vi "EV Rotator Initialize.vi"(0 "Run Step Inputs":T1={"Data in"=[], "Results in"=[], "Seq Setup in"="", "Step name"="", "Hardware in"="", "Calibration in"="", "Step # in sequence"=0, "Display step?(f)"=TRUE, "Generate names only"=FALSE, "Waveforms in"=[], "Memory List Grouping info"=[]} {"Waveforms in"."Y dB ref" format="%.1f"; "Waveforms in"."Y axis" items=["dB", "Lin", "Pwr"]; "Waveforms in"."Y data" items=["dB", "Lin", "Pwr"]; "Waveforms in"."X data" items=["dB", "Lin", "Pwr"]; "Data in"."Z data" items=["dB", "Lin", "Pwr"]; "Data in"."X data" items=["dB", "Lin", "Pwr"]; "Data in"."Y data" items=["dB", "Lin", "Pwr"]; "Data in"."Z dB ref" format="%.1f"; "Data in"."Z axis" items=["Log", "Lin"]; "Data in"."X dB ref" format="%.1f"; "Data in"."X axis" items=["Log", "Lin"]; "Data in"."Y axis" items=["Log", "Lin"]; "Data in"."Y dB ref" format="%.1f"; "Data in"."Curve"."z" format="%.2f"; "Data in"."Curve"."y" format="%.2f"; "Data in"."Curve"."x" format="%.2f"; "Results in"."Unit type" items=["dB", "Lin", "Pwr"]; "Results in"."Margin" format="%.2f"}, 11 "error in (no error)":errorcluster) -> (6 "Data out":T2 {"Z data" items=["dB", "Lin", "Pwr"]; "X data" items=["dB", "Lin", "Pwr"]; "Y data" items=["dB", "Lin", "Pwr"]; "Z dB ref" format="%.1f"; "Z axis" items=["Log", "Lin"]; "X dB ref" format="%.1f"; "X axis" items=["Log", "Lin"]; "Y axis" items=["Log", "Lin"]; "Y dB ref" format="%.1f"; "Curve"."z" format="%.2f"; "Curve"."y" format="%.2f"; "Curve"."x" format="%.2f"}, 8 "Results out":T5 {"Unit type" items=["dB", "Lin", "Pwr"]; "Margin" format="%.2f"}, 10 "Waveforms out":T7 {"Y dB ref" format="%.1f"; "Y axis" items=["dB", "Lin", "Pwr"]; "Y data" items=["dB", "Lin", "Pwr"]; "X data" items=["dB", "Lin", "Pwr"]}, 15 "error out":errorcluster)   [LabVIEW 2016]
uses:
  custom and Sc run Seq Sub VIs (x64).llb/data array.ctl
  custom and Sc run Seq Sub VIs (x64).llb/data cluster.ctl
  custom and Sc run Seq Sub VIs (x64).llb/Axis Unit Type.ctl
  custom and Sc run Seq Sub VIs (x64).llb/result array.ctl
  custom and Sc run Seq Sub VIs (x64).llb/result cluster.ctl
  custom and Sc run Seq Sub VIs (x64).llb/waveform array.ctl
  custom and Sc run Seq Sub VIs (x64).llb/waveform cluster.ctl
  custom and Sc run Seq Sub VIs (x64).llb/Run Step Inputs.ctl
  custom and Sc run Seq Sub VIs (x64).llb/Memory List Grouping.ctl
  custom and Sc run Seq Sub VIs (x64).llb/Memory List Grouping - Item Type.ctl
  custom and Sc run Seq Sub VIs (x64).llb/window stack manager Functions.ctl
  C:/SoundCheck 17/System/Custom VIs/EV.Rotator.RotatorControl.dll
  EV.Rotator.RotatorControl.dll
panel:
  # "NOTE:  These controls and indicators must stay here, but you can Hide them if you wish.  These are wired as the standard input/output connector pane for step run VIs."
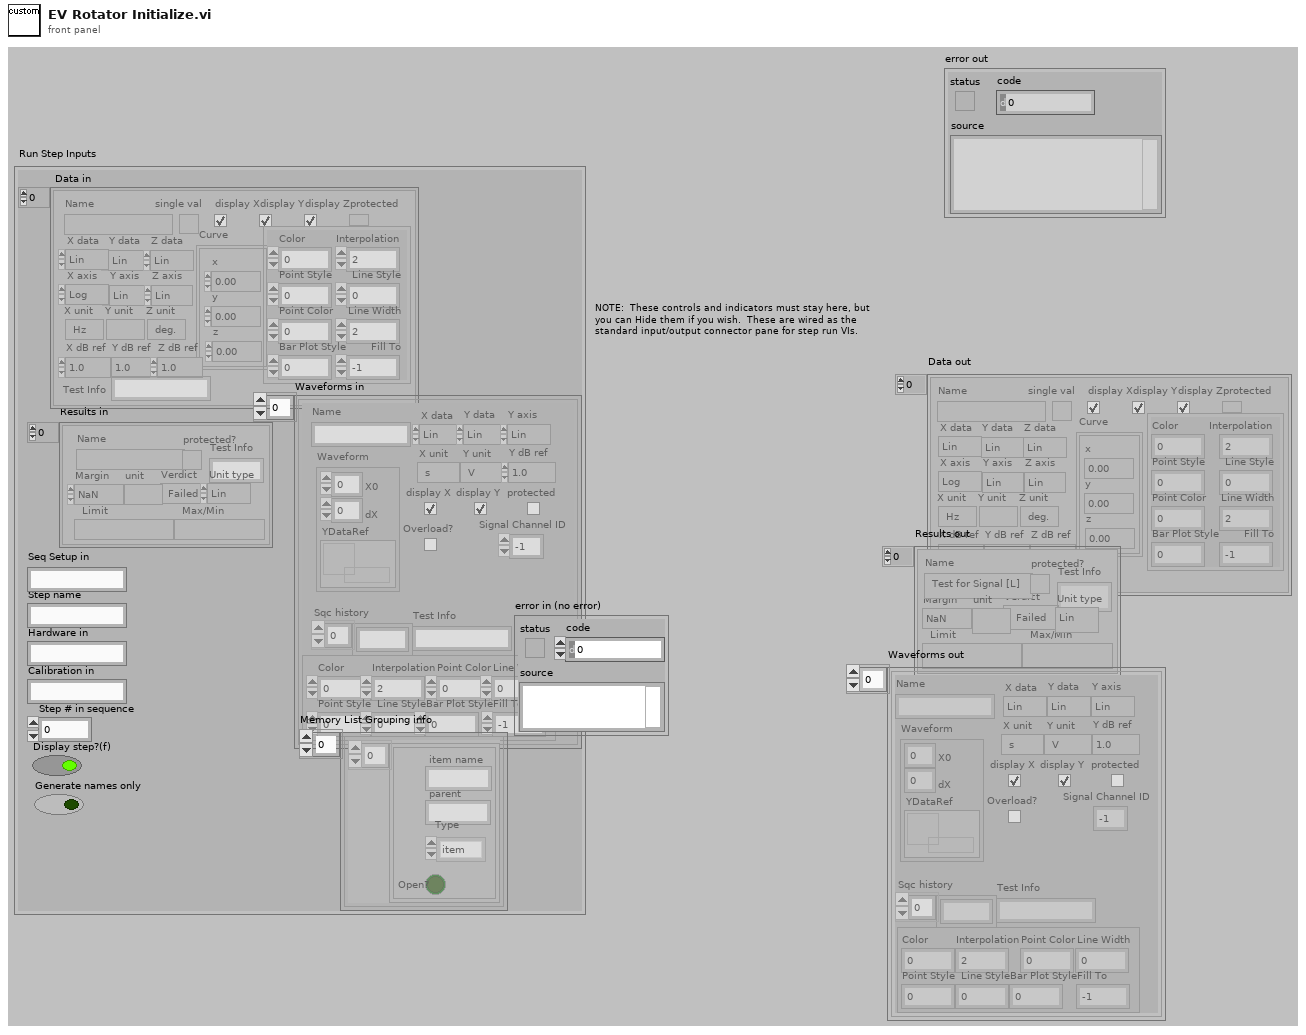
[diagram p1: front panel]
types:
  T1 = typedef "Run Step Inputs.ctl" = cluster{"Data in":T2, "Results in":T5, "Seq Setup in":string, "Step name":string, "Hardware in":string, "Calibration in":string, "Step # in sequence":i32, "Display step?(f)":bool, "Generate names only":bool, "Waveforms in":T7, "Memory List Grouping info":cluster{T9[]}[]}
  T2 = typedef "data array.ctl" = T3[]
  T3 = typedef "data cluster.ctl" = cluster{"Name":string, "Curve":cluster{"x":dbl, "y":dbl, "z":dbl}[], "X data":T4, "Y data":T4, "Z data":T4, "X axis":u16, "Y axis":u16, "Z axis":u16, "X unit":string, "Y unit":string, "Z unit":string, "X dB ref":dbl, "Y dB ref":dbl, "Z dB ref":dbl, "single val":bool, "protected":bool, "display X":bool, "display Y":bool, "display Z":bool, "Plot Settings":cluster{"Color":u32, "Interpolation":u8, "Point Style":u8, "Line Style":u8, "Point Color":u32, "Line Width":u8, "Bar Plot Style":u8, "Fill To":i16}, "Test Info":string}
  T4 = typedef "Axis Unit Type.ctl" = u16
  T5 = typedef "result array.ctl" = T6[]
  T6 = typedef "result cluster.ctl" = cluster{"Name":string, "Margin":dbl, "unit":string, "Verdict":bool, "Limit":string, "Max/Min":string, "protected?":bool, "Test Info":string, "Unit type":T4}
  T7 = typedef "waveform array.ctl" = T8[]
  T8 = typedef "waveform cluster.ctl" = cluster{"Name":string, "Waveform":cluster{"X0":dbl, "dX":dbl, "YDataRef":refnum<data-value>}, "X data":T4, "Y data":T4, "Y axis":T4, "X unit":string, "Y unit":string, "Y dB ref":dbl, "display Y":bool, "display X":bool, "Overload?":bool, "protected":bool, "Sqc history":string[], "Signal Channel ID":i32, "Plot Settings":cluster{"Color":u32, "Interpolation":u8, "Point Style":u8, "Line Style":u8, "Point Color":u32, "Line Width":u8, "Bar Plot Style":u8, "Fill To":i16}, "Test Info":string}
  T9 = typedef "Memory List Grouping.ctl" = cluster{"item name":string, "parent":string, "Open?":bool, "Type":T10}
  T10 = typedef "Memory List Grouping - Item Type.ctl" = enum16{"item", "custom group", "auto group", "protected group"}
  T11 = typedef "window stack manager Functions.ctl" = enum16{"Init", "add", "remove", "run", "clear", "vi stopped offset", "minimize all", "restore all", "autoadd", "Hourglass On", "Hourglass Off"}
  T12 = typedef "seq step setup.ctl" = cluster{"Input Signal Channels":i32[], "Output Signal Channels":i32[], "Curves selected":string[][], "Curves generated":string[], "Step setup flat":string, "Trigger Signal Channel":i32, "Curves Generated Assumptions":cluster{"seq-setup in":string, "Relevant subset of mem list Grouping":cluster{T9[]}[]}}
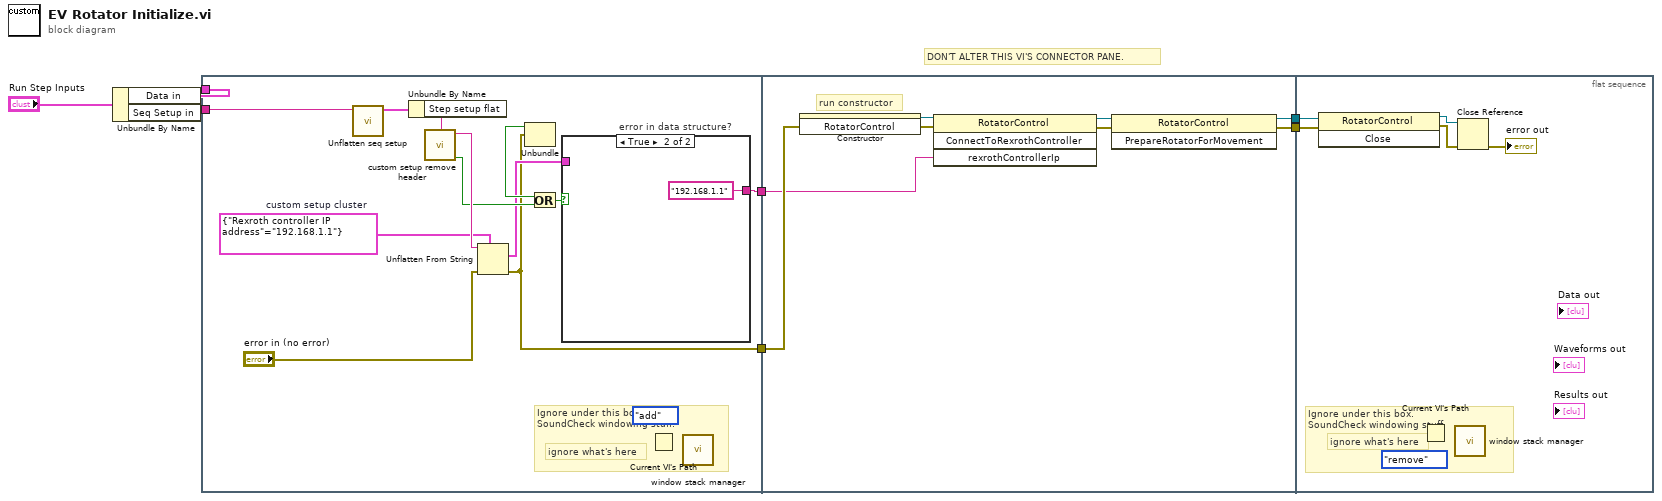
[diagram p0: block diagram]
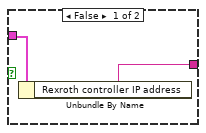
[diagram p2: hidden frame]
diagram:
  # "DON'T ALTER THIS VI'S CONNECTOR PANE."
  n1 = Unbundle By Name("Run Step Inputs") -> ("Data in"=w5:T2, "Seq Setup in"=w4:string)
  n2 = flat-sequence {
    tunnel: w5 -> [_]
    tunnel: w4 -> [w13]
    tunnel: [w12] -> w6
    tunnel: [w9] -> w3
    tunnel: w6 -> [w31]
    tunnel: w3 -> [w32]
    tunnel: [w28] -> w2
    tunnel: [w27] -> w1
    tunnel: w2 -> [w34]
    tunnel: w1 -> [w33]
    frame #0 {
      w8 = cluster{"Rexroth controller IP address":string} {"Rexroth controller IP address"="192.168.1.1"}  # custom setup cluster
      # "Ignore under this box. \nSoundCheck windowing stuff."
      # "ignore what's here"
      n3 = call "Unflatten seq setup.vi"("Unflatten seq setup"=w13) -> ("Sequence-specific step set-up"=w21:T12)  [unwired: 3 in, 7 out]
      n4 = Unbundle By Name(w21) -> ("Step setup flat"=w20:string)
      n5 = call "custom setup remove header.vi"("Output from 'Step setup flat' of seq-setup structure"=w20) -> ("Error?"=w18:bool, "Flattened custom step setup cluster"=w19:string)  [unwired: 9 out]
      n6 = Unflatten From String(type=w8, binary string=w19, error in (no error)="error in (no error)") -> (value=w15:cluster{"Rexroth controller IP address":string}, error out=w9:errorcluster)  [unwired: 3 out]
      n7 = Unbundle(w9) -> ("status"=w17:bool)  [unwired: 2 out]
      n8 = Or(x=w17, y=w18) -> (x .or. y?=w16:bool)
      n9 = case "error in data structure?" shown="True" w16 {
        tunnel: [w23 "192.168.1.1" ("Rexroth controller IP address")] -> w12
        tunnel: w15 -> [w22 _]
        frame False {
          n10 = Unbundle By Name(w22) -> ("Rexroth controller IP address"=w23:string)
        }
        frame True {
        }
      }
      n11 = Current VI's Path() -> (path=w14:path)
      n12 = call "window stack manager.vi"("VI path"=w14, "Function (run)"=window_stack_manager_Functions."add") -> ()  [unwired: 5 in, 5 out]
    }
    frame #1 {
      # "run constructor"
      n13 = constructor class="RotatorControl"(error in=w32) -> (reference out=w26:refnum<k24>, error out=w25:errorcluster)  [unwired: 2 in, 1 out]
      n14 = invoke class="RotatorControl" method="ConnectToRexrothController"(reference=w26, error in=w25, "rexrothControllerIp"=w31) -> (reference out=w30:refnum<k24>, error out=w29:errorcluster)  [unwired: 1 in, 2 out]
      n15 = invoke class="RotatorControl" method="PrepareRotatorForMovement"(reference=w30, error in=w29) -> (reference out=w28:refnum<k24>, error out=w27:errorcluster)  [unwired: 1 in, 1 out]
    }
    frame #2 {
      # "Ignore under this box. \nSoundCheck windowing stuff."
      # "ignore what's here"
      n16 = invoke class="RotatorControl" method="Close"(reference=w34, error in=w33) -> (reference out=w35:refnum<k24>, error out=w36:errorcluster)  [unwired: 1 in, 1 out]
      n17 = Current VI's Path() -> (path=w39:path)
      n18 = call "window stack manager.vi"("VI path"=w39, "Function (run)"=window_stack_manager_Functions."remove") -> ()  [unwired: 5 in, 5 out]
      n19 = Close Reference(reference=w35, error in (no error)=w36) -> (error out=→"error out":errorcluster)
    }
  }
